vi "to string.vi"(8 "error in":errorcluster, 11 "fixed channel configuration in":refnum<class "control module configuration.lvclass">) -> (0 "error out":errorcluster, 1 "data":string, 2 "version":string, 3 "fixed channel configuration out":refnum<class "control module configuration.lvclass">)   [LabVIEW 2013, in "control module configuration.lvclass"]
doc: "Provides an interface for saving a module configuration to a file or other serialized data source. It is recommended that all children of this class store data in two sets--data required for its own initialization, and any data required for parent initialization--and that each implementation uses the <b>Call Parent Method</b> primitive to serialize parent information.\nNI Tag Bus Module Framework 1.0.3.43\nNI Systems Engineering"
uses:
  control module configuration.lvclass
  <vilib>/NI/Tag Bus Module Framework/module configuration/TBM module configuration.lvclass
  control module configuration.lvclass/control module configuration.ctl
  <vilib>/NI/Tag Bus Module Framework/channel/TBM channel.lvclass
  <vilib>/NI/Configuration Framework/serializable configuration/NISE_CEF_serializable configuration.lvclass
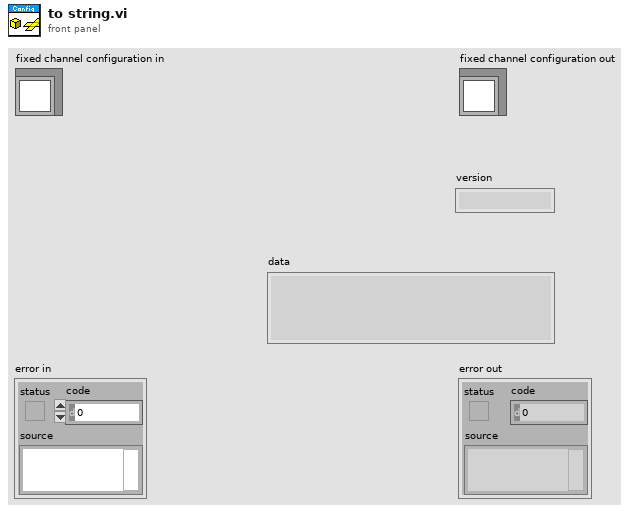
[diagram p1: front panel]
types:
  T1 = typedef "control module configuration.lvclass/error classification.ctl" = cluster{"code":i32, "error classification":T2}
  T2 = typedef "TBM module execution interface.lvclass/error classification.ctl" = enum16{"unknown", "none", "trivial", "recoverable", "critical"}
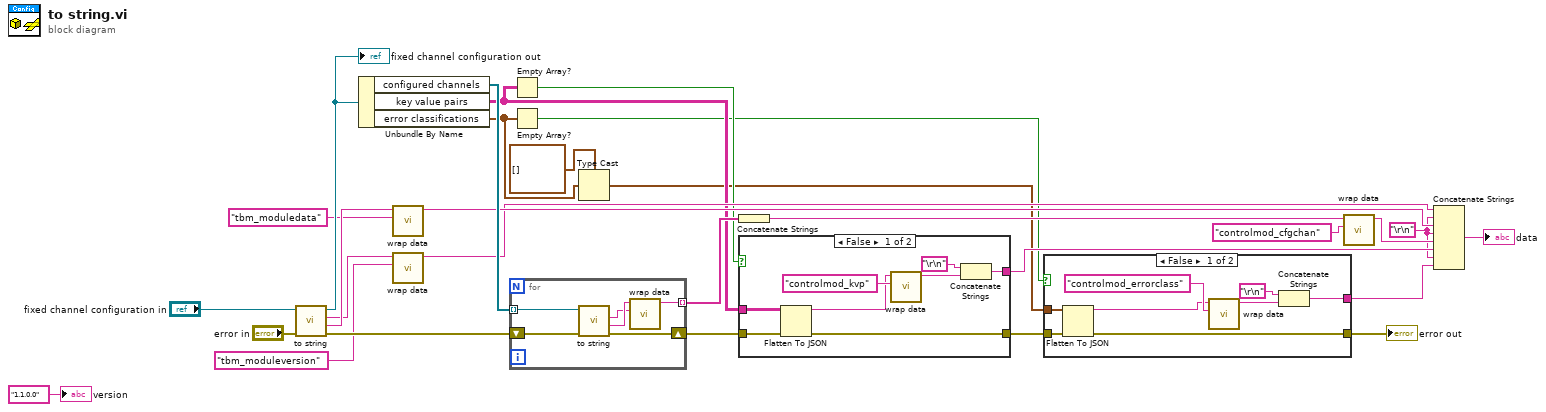
[diagram p0: block diagram]
diagram:
  w5 = "\r\n"
  n1 = call-parent "to string.vi"("error in"="error in", "module configuration in"="fixed channel configuration in") -> ("error out"=w25:errorcluster, "data"=w16:string, "version"=w15:string, "module configuration out"=w27:refnum<class "control module configuration.lvclass">)  [unwired: 6 in]
  "fixed channel configuration out" <- w27
  n2 = Unbundle By Name(w27) -> ("configured channels"=w24:refnum<class "TBM channel.lvclass">[], "key value pairs"=w10:string[][], "error classifications"=w3:T1[])
  n3 = call <vilib>:"wrap data.vi"("identifier"="tbm_moduledata", "data to wrap"=w16) -> ("wrapped data"=w18:string)  [unwired: 9 in]
  n4 = call <vilib>:"wrap data.vi"("identifier"="tbm_moduleversion", "data to wrap"=w15) -> ("wrapped data"=w17:string)  [unwired: 9 in]
  n5 = for {
    tunnel: w24 -> [w35] mode=indexing
    shift-right: [w31] -> w9
    shift-left: w25 -> [w32]
    tunnel: [w30] -> w20 mode=indexing
    n6 = call-dynamic "to string.vi"("error in"=w32, "channel in"=w35) -> ("error out"=w31:errorcluster, "channel data"=w34:string, "identifier"=w33:string)  [unwired: 6 in, 1 out]
    n7 = call <vilib>:"wrap data.vi"("identifier"=w33, "data to wrap"=w34) -> ("wrapped data"=w30:string)  [unwired: 9 in]
  }
  n8 = Empty Array?(array=w10) -> (empty?=w11:bool)
  n9 = Empty Array?(array=w3) -> (empty?=w4:bool)
  n10 = Type Cast(type=cluster{i32, i32}[] [], x=w3) -> (*(type *) &x=w1:cluster{i32, i32}[])
  n11 = Concatenate Strings(w20) -> (w19:string)
  n12 = case shown="False" w11 {
    tunnel: [w41 _] -> w12
    tunnel: w10 -> [w38 _]
    tunnel: w9 -> [w39 w44]
    tunnel: [w36 w44] -> w8
    frame False {
      n13 = Flatten To JSON(anything=w38, error in (no error)=w39) -> (JSON string=w37:string, 11:w36:errorcluster)  [unwired: 1 in]
      n14 = call <vilib>:"wrap data.vi"("identifier"="controlmod_kvp", "data to wrap"=w37) -> ("wrapped data"=w42:string)  [unwired: 9 in]
      n15 = Concatenate Strings("\r\n", w42) -> (w41:string)
    }
    frame True {
    }
  }
  n16 = case shown="False" w4 {
    tunnel: [w50 _] -> w6
    tunnel: w1 -> [w47 _]
    tunnel: w8 -> [w48 w53]
    tunnel: [w45 w53] -> w7
    frame False {
      n17 = Flatten To JSON(anything=w47, error in (no error)=w48) -> (JSON string=w46:string, 11:w45:errorcluster)  [unwired: 1 in]
      n18 = call <vilib>:"wrap data.vi"("identifier"="controlmod_errorclass", "data to wrap"=w46) -> ("wrapped data"=w51:string)  [unwired: 9 in]
      n19 = Concatenate Strings("\r\n", w51) -> (w50:string)
    }
    frame True {
    }
  }
  "error out" <- w7
  n20 = call <vilib>:"wrap data.vi"("identifier"="controlmod_cfgchan", "data to wrap"=w19) -> ("wrapped data"=w23:string)  [unwired: 9 in]
  n21 = Concatenate Strings(w17, w5, w18, w5, w23, w12, w5, w6) -> (→"data":string)
  "version" <- "1.1.0.0" ("version")
